vi "111_IO.vi"() -> ()   [LabVIEW 2020]
uses:
  Libraries/S7/S7.lvlib
panel:
  in  "选项卡控件":enum32{"数字量输入", "数字量输出", "模拟量/伺服"}(tab)
  out "I 0":T1
  out "I 1":T2
  out "I 2":T3
  out "I 3":T4
  in  "Q 2":T5
  in  "Q 0":T6
  in  "Q 1":T7
  in  "Q 3":T8
  # "上下柱管压装"
  # "/"
  # "蜗杆伺服"
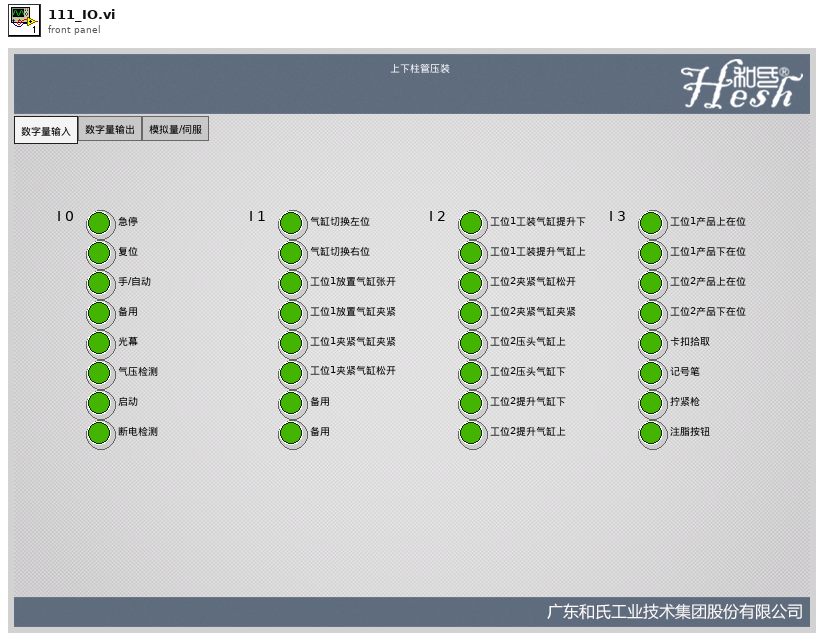
[diagram p1: front panel]
types:
  T1 = cluster{"急停":bool, "复位":bool, "手/自动":bool, "备用":bool, "光幕":bool, "气压检测":bool, "启动":bool, "断电检测":bool}
  T2 = cluster{"气缸切换左位":bool, "气缸切换右位":bool, "工位1放置气缸张开":bool, "工位1放置气缸夹紧":bool, "工位1夹紧气缸夹紧":bool, "工位1夹紧气缸松开":bool, "备用":bool, "备用":bool}
  T3 = cluster{"工位1工装气缸提升下":bool, "工位1工装提升气缸上":bool, "工位2夹紧气缸松开":bool, "工位2夹紧气缸夹紧":bool, "工位2压头气缸上":bool, "工位2压头气缸下":bool, "工位2提升气缸下":bool, "工位2提升气缸上":bool}
  T4 = cluster{"工位1产品上在位":bool, "工位1产品下在位":bool, "工位2产品上在位":bool, "工位2产品下在位":bool, "卡扣拾取":bool, "记号笔":bool, "拧紧枪":bool, "注脂按钮":bool}
  T5 = cluster{bool, bool, bool, bool, "工位1夹紧气缸夹紧":bool, "工位1夹紧气缸松开":bool, "工位1提升气缸下降":bool, "工位1提升气缸上升":bool}
  T6 = cluster{"/":bool, "/":bool, "/":bool, "/":bool, "蜂鸣器":bool, "黄灯":bool, "绿灯":bool, "红灯":bool}
  T7 = cluster{"OK指示灯":bool, "NG指示灯":bool, bool, bool, "/":bool, "/":bool, "/":bool, "/":bool}
  T8 = cluster{bool, bool, bool, bool, "工位2提升气缸下降":bool, "工位2提升气缸上升":bool, "/":bool, "/":bool}
  T9 = cluster{bool, bool, bool, bool, bool, bool, bool, bool}
  T10 = cluster{"[0]":bool, "[1]":bool, "[2]":bool, "[3]":bool, "[4]":bool, "[5]":bool, "[6]":bool, "[7]":bool}
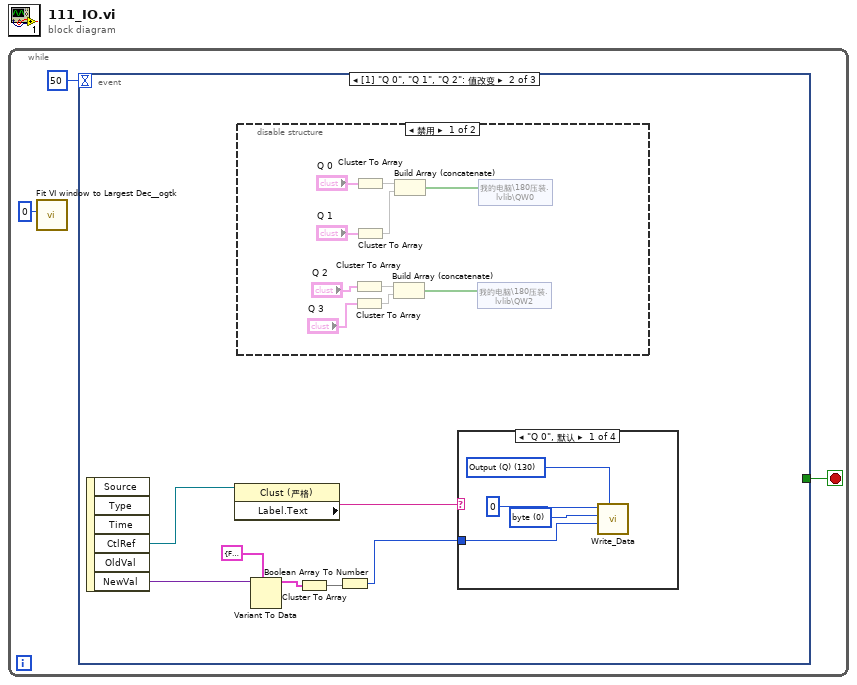
[diagram p0: block diagram]
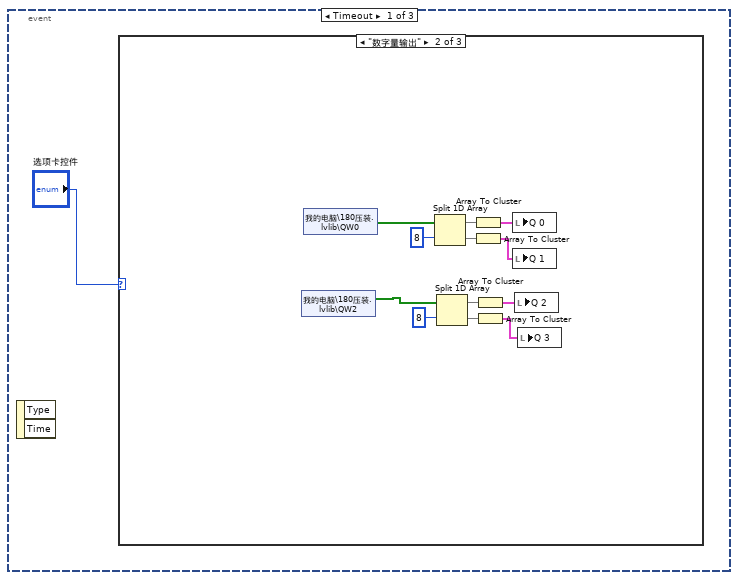
[diagram p2: hidden frame]
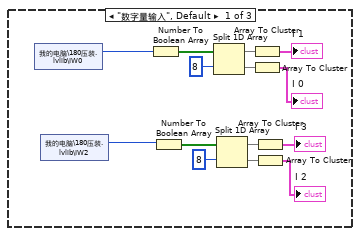
[diagram p3: hidden frame]
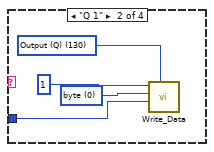
[diagram p6: hidden frame]
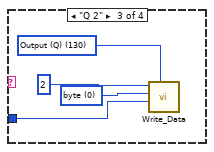
[diagram p7: hidden frame]
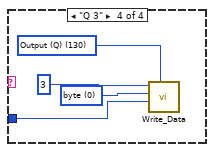
[diagram p8: hidden frame]
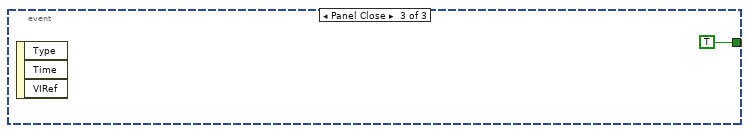
[diagram p9: hidden frame]
diagram:
  n1 = while {
    stop <- w3 stop-if-true
    n2 = call <userlib>:"Fit VI window to Largest Dec__ogtk.vi"("border spacing (2 px)"=0) -> ()  [unwired: 5 in, 2 out]
    n3 = event shown="[1] \"Q 0\", \"Q 1\", \"Q 2\": 值改变" {
      selector: _ -> [_ _ _]
      dyn-events: _ -> [_ _ _]
      timeout: 50 -> [_ _ _]
      tunnel: [_ _ TRUE] -> w3
      event Timeout {
        n4 = event-data() -> ()  [unwired: 1 in, 2 out]
        n5 = case shown="\"数字量输出\"" "选项卡控件" {
          frame "数字量输入", Default {
            n6 = shared-variable "我的电脑\\180压装.lvlib\\IW0"() -> (w8:u16)  [unwired: 1 in, 1 out]
            n7 = shared-variable "我的电脑\\180压装.lvlib\\IW2"() -> (w7:u16)  [unwired: 1 in, 1 out]
            n8 = Number To Boolean Array(number=w8) -> (Boolean array=w18:bool[])
            n9 = Number To Boolean Array(number=w7) -> (Boolean array=w17:bool[])
            n10 = Split 1D Array(array=w18, index=8 ("索引")) -> (first subarray=w16:bool[], second subarray=w13:bool[])
            n11 = Split 1D Array(array=w17, index=8 ("索引")) -> (first subarray=w14:bool[], second subarray=w15:bool[])
            n12 = Array To Cluster(array=w16) -> (cluster=→"I 1":T10)
            n13 = Array To Cluster(array=w13) -> (cluster=→"I 0":T10)
            n14 = Array To Cluster(array=w14) -> (cluster=→"I 3":T10)
            n15 = Array To Cluster(array=w15) -> (cluster=→"I 2":T10)
          }
          frame "数字量输出" {
            n16 = shared-variable "我的电脑\\180压装.lvlib\\QW2"() -> (w21:bool[])  [unwired: 1 in, 1 out]
            n17 = shared-variable "我的电脑\\180压装.lvlib\\QW0"() -> (w22:bool[])  [unwired: 1 in, 1 out]
            n18 = Split 1D Array(array=w22, index=8 ("索引")) -> (first subarray=w30:bool[], second subarray=w29:bool[])
            n19 = Split 1D Array(array=w21, index=8 ("索引")) -> (first subarray=w24:bool[], second subarray=w25:bool[])
            n20 = Array To Cluster(array=w30) -> (cluster=w28:T10)
            n21 = Array To Cluster(array=w29) -> (cluster=w27:T10)
            n22 = Array To Cluster(array=w24) -> (cluster=w26:T10)
            n23 = Array To Cluster(array=w25) -> (cluster=w23:T10)
            n24 = local write "Q 0"(w28) -> ()
            n25 = local write "Q 1"(w27) -> ()
            n26 = local write "Q 2"(w26) -> ()
            n27 = local write "Q 3"(w23) -> ()
          }
          frame "模拟量/伺服" {
          }
        }
      }
      event "Q 0", "Q 1", "Q 2": Value Change {
        n28 = event-data() -> ("CtlRef"=w37:refnum<vi>, "NewVal"=w35:variant)  [unwired: 1 in, 4 out]
        n29 = property class="Clust (严格)"(reference=w37) -> ("Label.Text"=w36:string)  [unwired: 1 in, 2 out]
        n30 = disable-structure shown="禁用" {
          frame Disabled {
            n31 = Cluster To Array(cluster="Q 2") -> (array=w43:bool[])
            n32 = Cluster To Array(cluster="Q 3") -> (array=w41:bool[])
            n33 = Cluster To Array(cluster="Q 0") -> (array=w45:bool[])
            n34 = Cluster To Array(cluster="Q 1") -> (array=w44:bool[])
            n35 = Build Array (concatenate)(w43, w41) -> (w39:bool[])
            n36 = Build Array (concatenate)(w45, w44) -> (w38:bool[])
            n37 = shared-variable "我的电脑\\180压装.lvlib\\QW2"(w39) -> ()  [unwired: 1 in, 1 out]
            n38 = shared-variable "我的电脑\\180压装.lvlib\\QW0"(w38) -> ()  [unwired: 1 in, 1 out]
          }
          frame Enabled {
          }
        }
        n39 = Variant To Data(type=T9 {FALSE, FALSE, FALSE, FALSE, FALSE, FALSE, FALSE, FALSE}, Variant=w35) -> (data=w32:T9)  [unwired: 1 in, 1 out]
        n40 = Cluster To Array(cluster=w32) -> (array=w31:bool[])
        n41 = Boolean Array To Number(Boolean array=w31) -> (number=w33:u32)
        n42 = case shown="\"Q 0\", 默认" w36 {
          tunnel: w33 -> [w48 w52 w56 w60]
          frame "Q 0", Default {
            w49 = u16 0 items=["byte", "word", "Dword"] ("数据类型")
            w51 = u8 130 items=["I/O (P)"=128, "Input (I)"=129, "Output (Q)"=130, "Bit Memory (M)"=131, "Data (DB)"=132, "Instance Data (DI)"=133, "Local Data (L)"=134, "Predecessor Local Data (VL)"=135] ("寄存器类型")
            n43 = call "Write_Data.vi"("寄存器类型"=w51, "写入数据"=w48, "数据类型"=w49, "写入地址"=u32 0) -> ()  [unwired: 5 in, 3 out]
          }
          frame "Q 1" {
            w53 = u16 0 items=["byte", "word", "Dword"] ("数据类型")
            w55 = u8 130 items=["I/O (P)"=128, "Input (I)"=129, "Output (Q)"=130, "Bit Memory (M)"=131, "Data (DB)"=132, "Instance Data (DI)"=133, "Local Data (L)"=134, "Predecessor Local Data (VL)"=135] ("寄存器类型")
            n44 = call "Write_Data.vi"("寄存器类型"=w55, "写入数据"=w52, "数据类型"=w53, "写入地址"=u32 1) -> ()  [unwired: 5 in, 3 out]
          }
          frame "Q 2" {
            w57 = u16 0 items=["byte", "word", "Dword"] ("数据类型")
            w59 = u8 130 items=["I/O (P)"=128, "Input (I)"=129, "Output (Q)"=130, "Bit Memory (M)"=131, "Data (DB)"=132, "Instance Data (DI)"=133, "Local Data (L)"=134, "Predecessor Local Data (VL)"=135] ("寄存器类型")
            n45 = call "Write_Data.vi"("寄存器类型"=w59, "写入数据"=w56, "数据类型"=w57, "写入地址"=u32 2) -> ()  [unwired: 5 in, 3 out]
          }
          frame "Q 3" {
            w61 = u16 0 items=["byte", "word", "Dword"] ("数据类型")
            w63 = u8 130 items=["I/O (P)"=128, "Input (I)"=129, "Output (Q)"=130, "Bit Memory (M)"=131, "Data (DB)"=132, "Instance Data (DI)"=133, "Local Data (L)"=134, "Predecessor Local Data (VL)"=135] ("寄存器类型")
            n46 = call "Write_Data.vi"("寄存器类型"=w63, "写入数据"=w60, "数据类型"=w61, "写入地址"=u32 3) -> ()  [unwired: 5 in, 3 out]
          }
        }
      }
      event Panel Close {
        n47 = event-data() -> ()  [unwired: 1 in, 3 out]
      }
    }
  }
